vi "sort cycle unknown.vi"(6 "which order":string[](array[string])=["sequence number", "position", "seq total count", "seq total q", "seq unnormed ratio", "std total count", "std total pq", "std norm", "seq ratio", "seq ext error", "seq ext error(%)", "seq int error", "seq int error(%)", "seq error", "seq error(%)", "seq ext vs int"], 8 "error in":errorcluster) -> (0 "error out":errorcluster)   [LabVIEW 2016]
doc: "Takes a sample type and sorts by sequence"
uses:
  controls/data control cluster.ctl
  <vilib>/Analysis/baseanly.llb/Mean (DBL).vi
  <vilib>/Analysis/NI_AALBase.lvlib
panel:
  out "array w/ subset deleted":dbl[][][](array[numeric])
  out "cycle result header":string[](array[string])
  out "output array 2":dbl[][](array[numeric])
  out "element 2":i32
  out "output array":dbl[][](array[numeric])
  out "element":i32
  out "x/y 2":dbl
  out "x/y":dbl
  out "Cycle data by seq 4":dbl[][](array[numeric])
  out "Cycle data by seq 3":dbl[][](array[numeric])
  out "Array 3":bool[](array[boolean])
  out "Cycle data by seq 2":dbl[][][](array[numeric])
  out "DATA CLUSTER out 2":T1
  out "cycle results labels":string[](array[string])
  out "sequence result header 2":string[](array[string])
  out "Array 2":dbl[][](array[numeric])
  out "index of element":i32
  out "sequence  Result":dbl[][][](array[numeric])
  out "Final result header":string[][](array[string])
  out "DATA CLUSTER out":T1
  out "sequence result header":string[](array[string])
  out "Array":i32[](array[numeric])
  out "cycle results dbl 2":dbl[][](array[numeric])
  out "Cycle data by seq":dbl[][][](array[numeric])
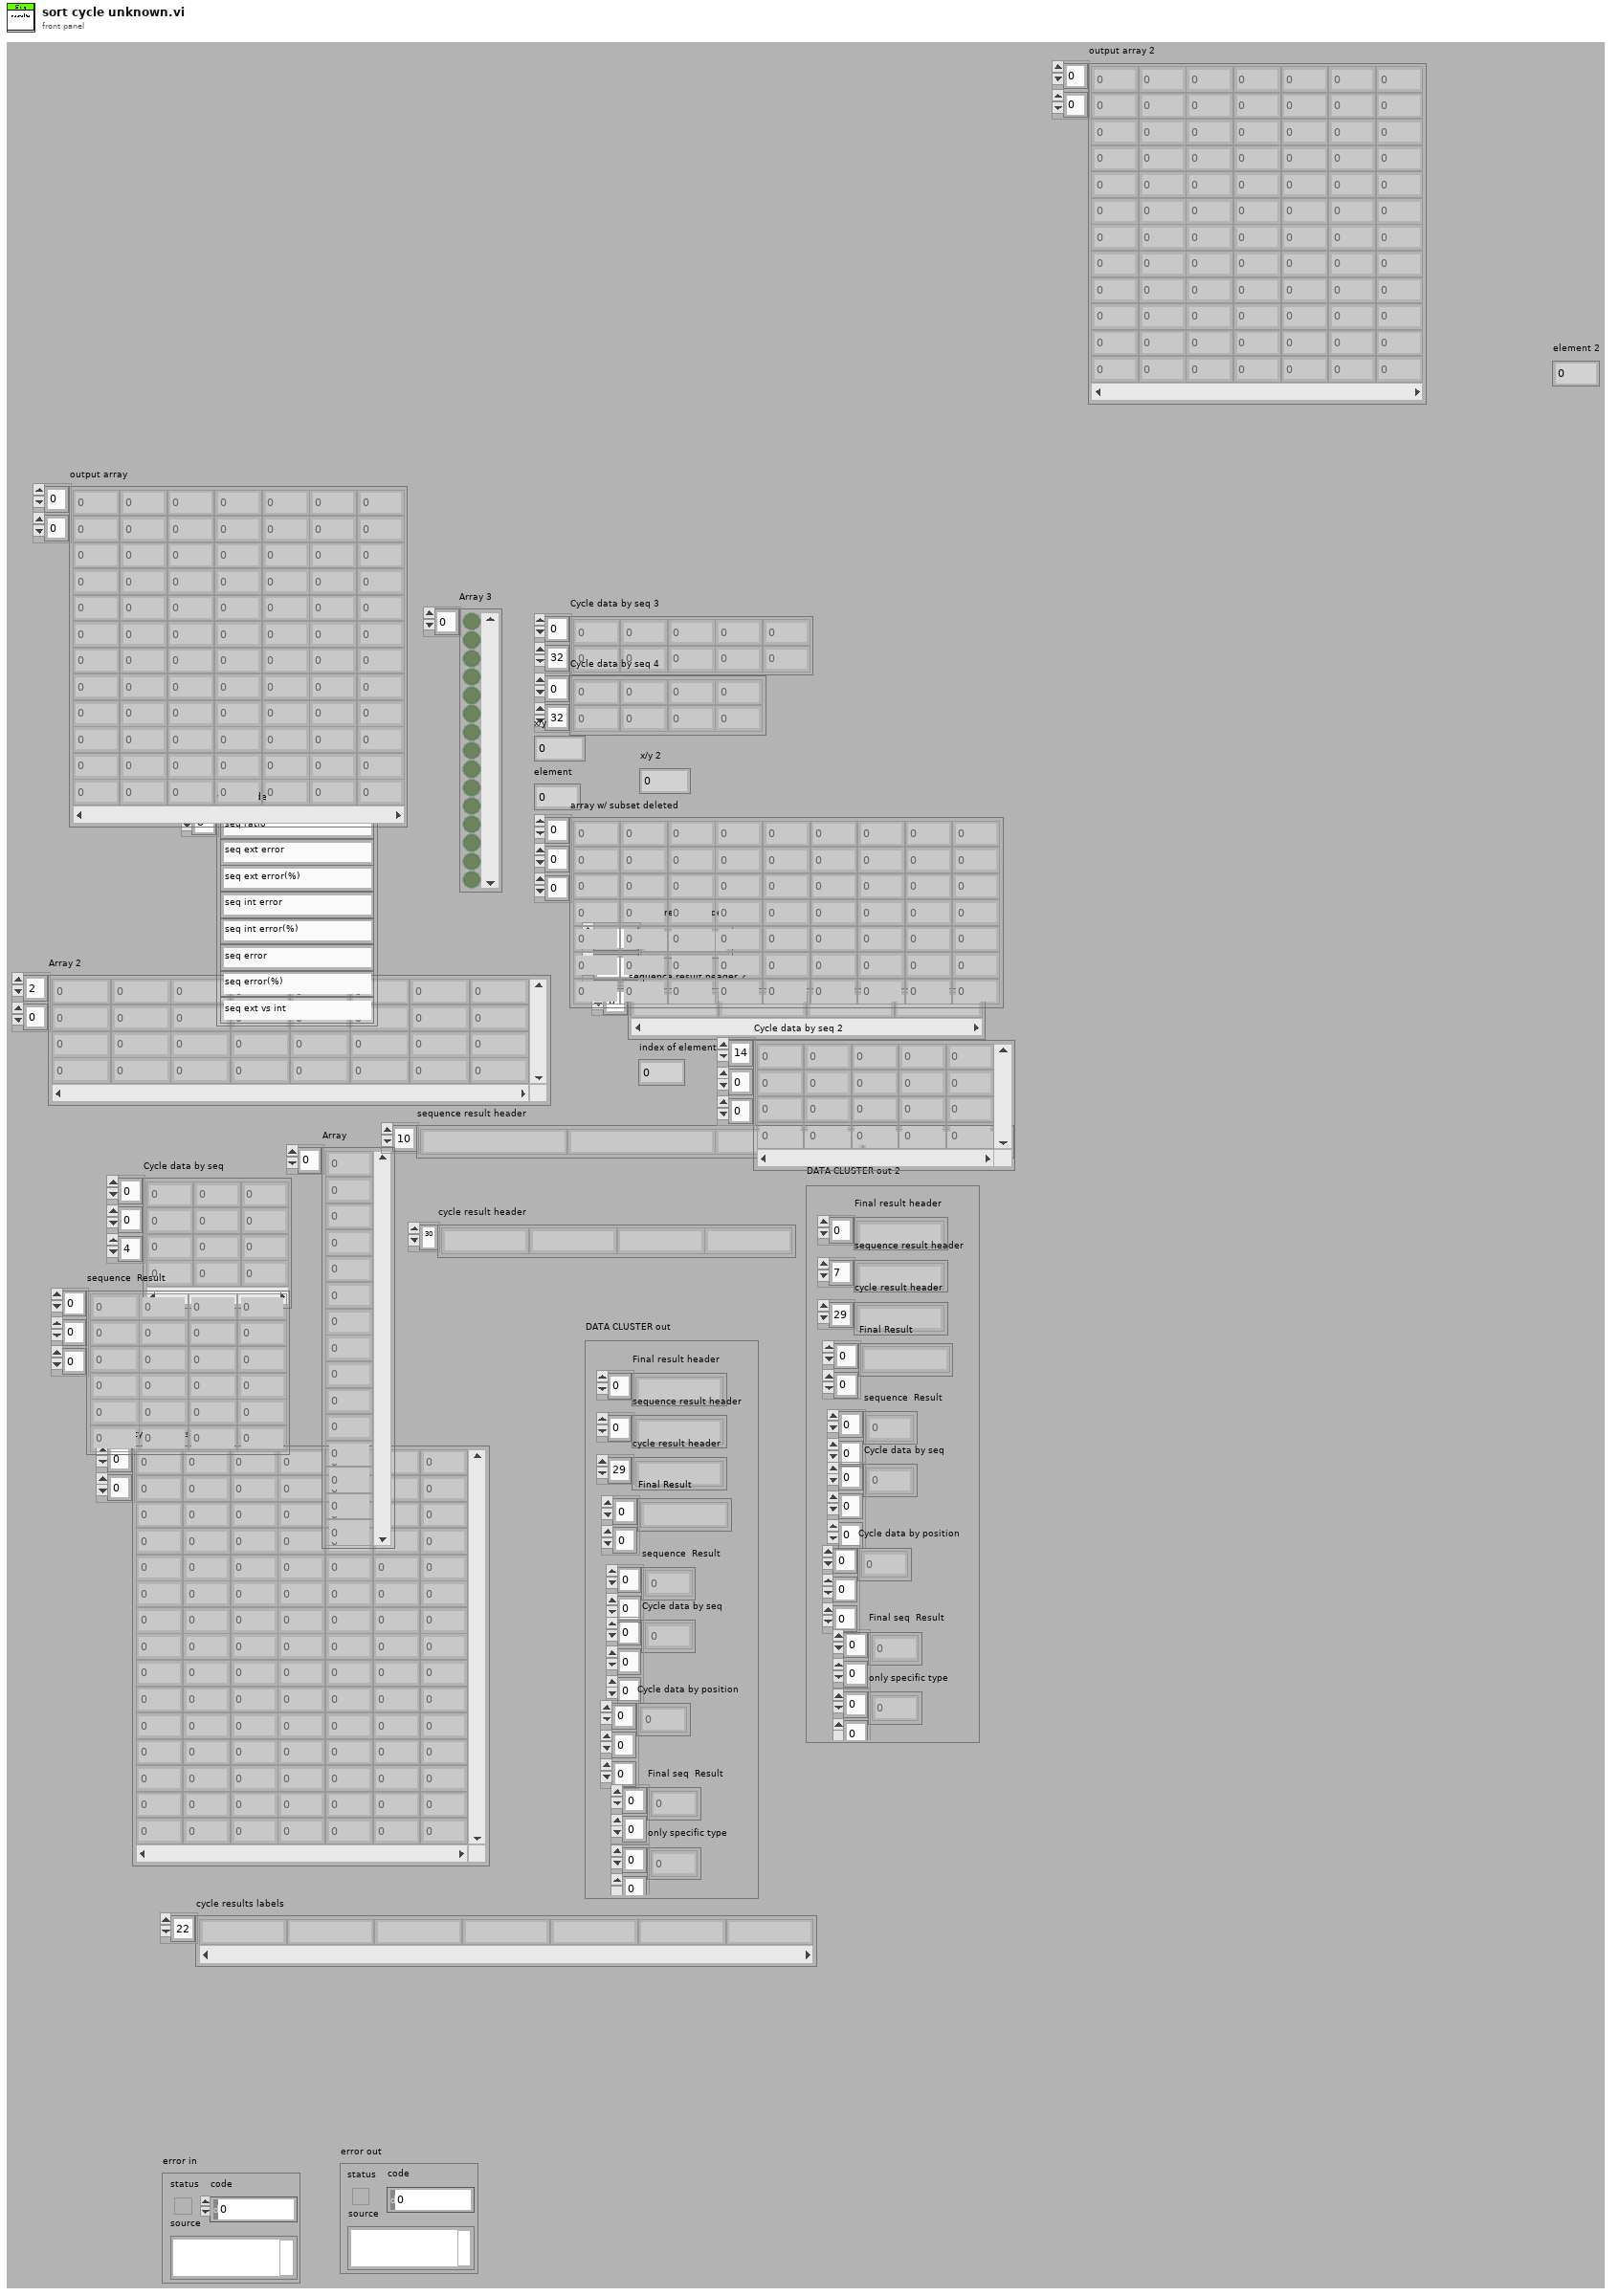
[diagram p1: front panel]
types:
  T1 = typedef "data control cluster.ctl" = cluster{"Final result header":string[], "sequence result header":string[], "cycle result header ":string[], "Final Result":string[][], "sequence  Result":dbl[][], "Cycle data by seq":dbl[][][], "Cycle data by position":dbl[][][], "Final seq  Result":dbl[][], "only specific type":dbl[][]}
  T2 = typedef "cycle results control.ctl" = cluster{"sample info":string[][], "cycle results labels":string[], "cycle results dbl":dbl[][]}
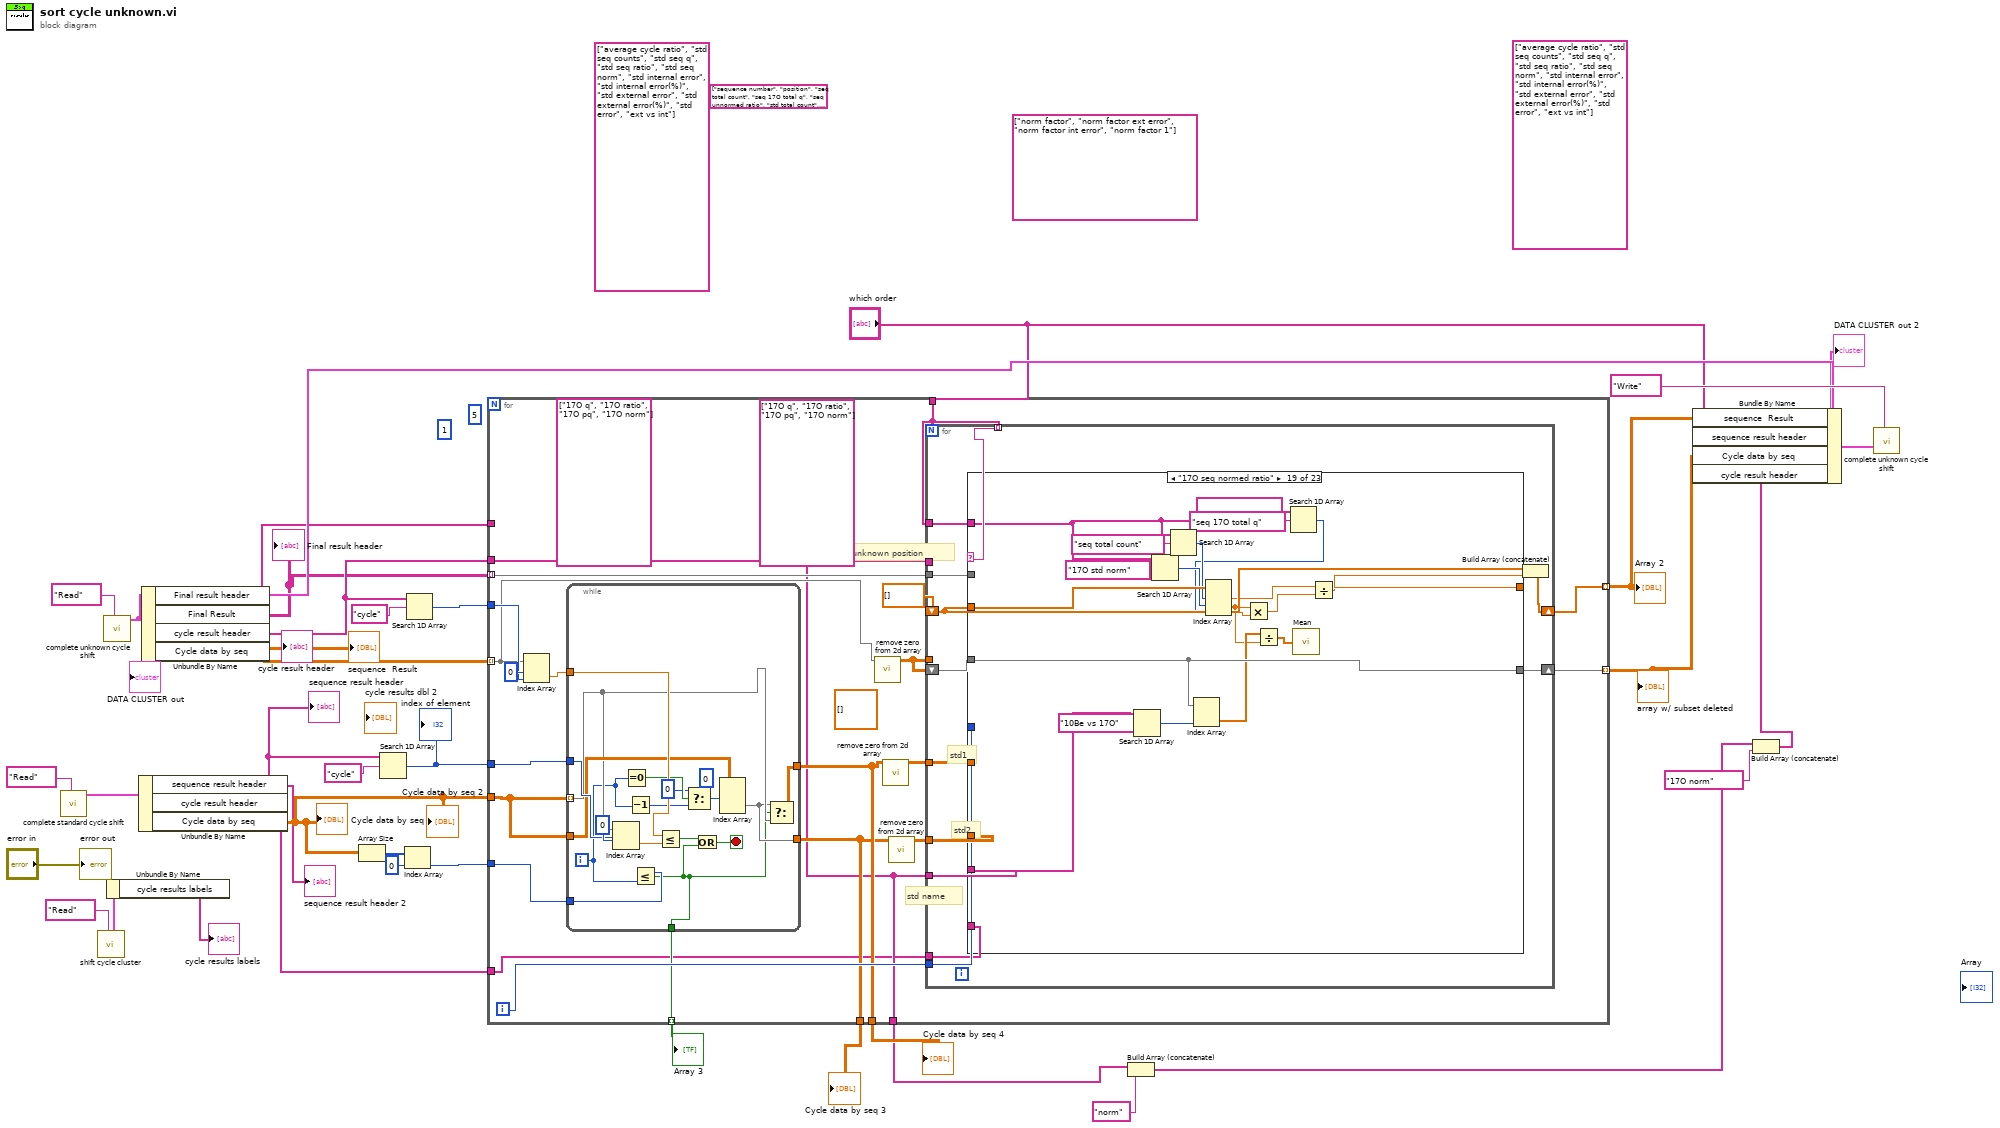
[diagram p0: block diagram]
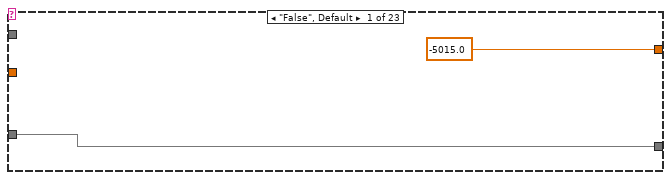
[diagram p2: hidden frame]
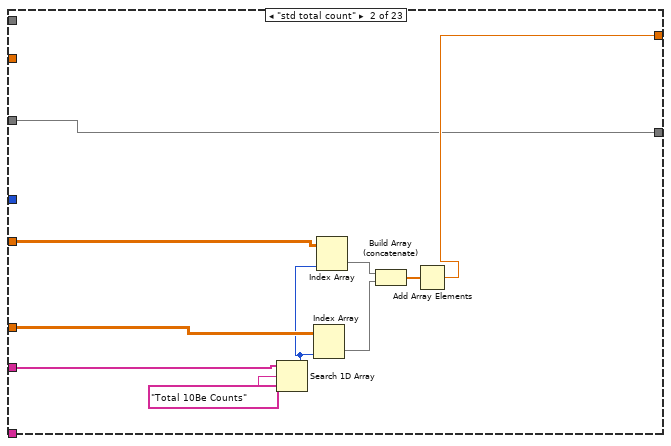
[diagram p3: hidden frame]
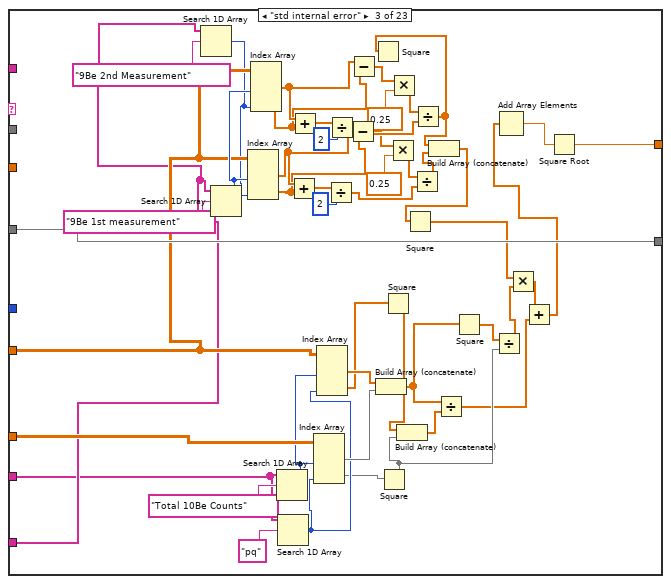
[diagram p4: hidden frame]
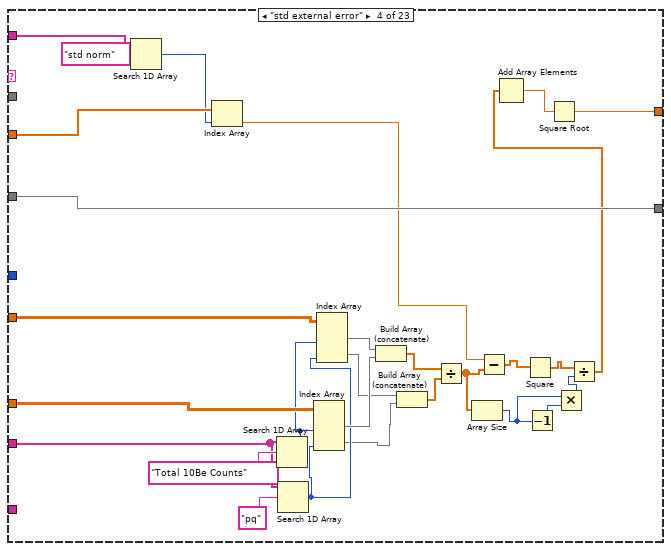
[diagram p5: hidden frame]
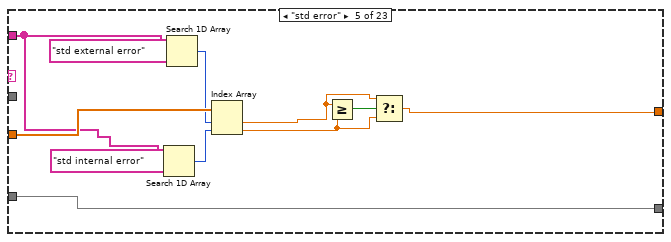
[diagram p6: hidden frame]
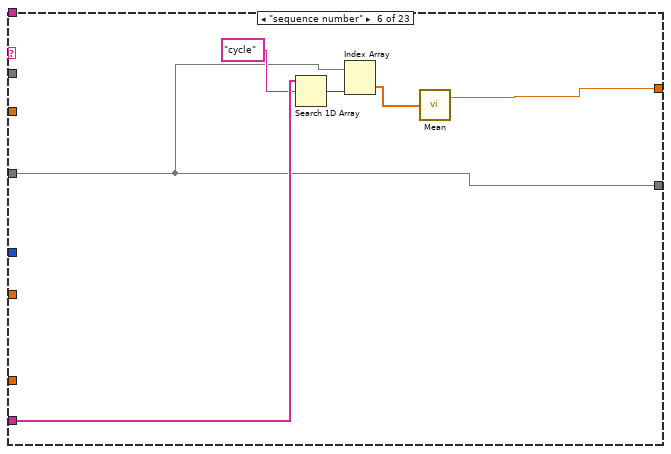
[diagram p7: hidden frame]
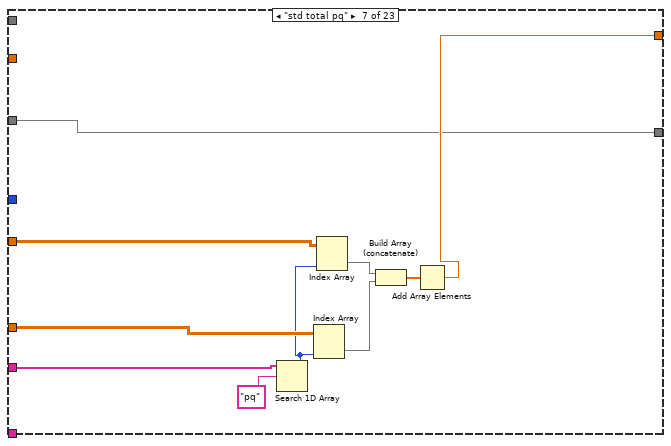
[diagram p8: hidden frame]
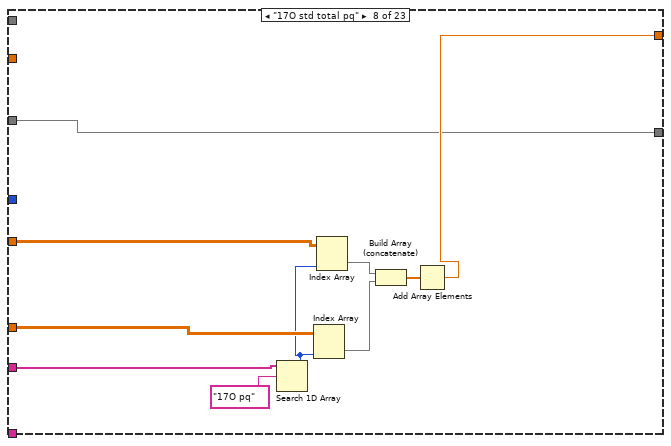
[diagram p9: hidden frame]
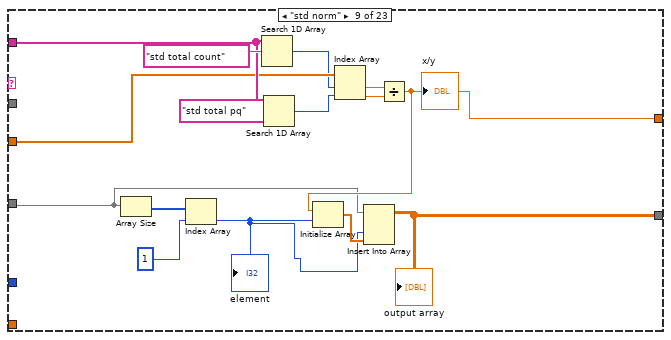
[diagram p10: hidden frame]
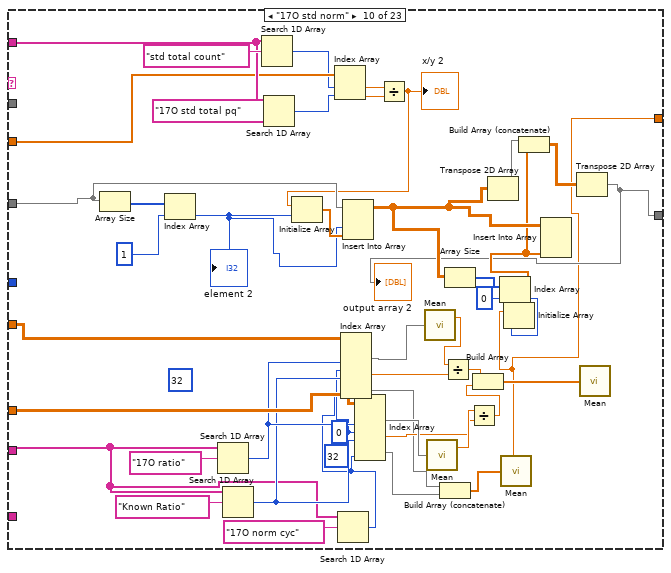
[diagram p11: hidden frame]
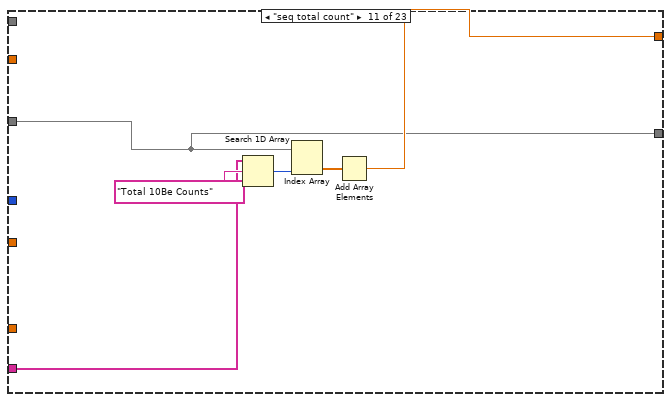
[diagram p12: hidden frame]
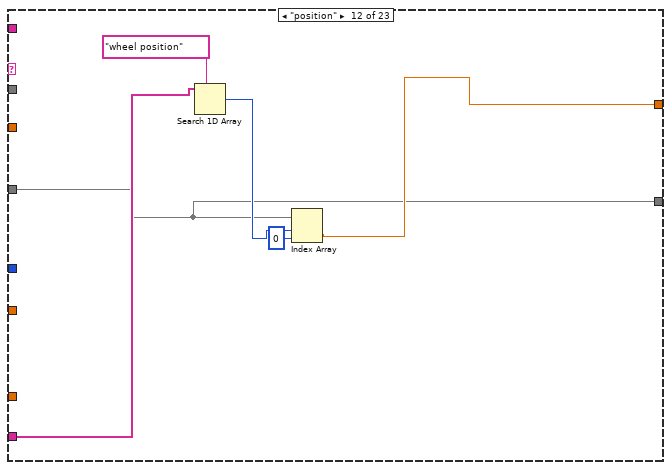
[diagram p13: hidden frame]
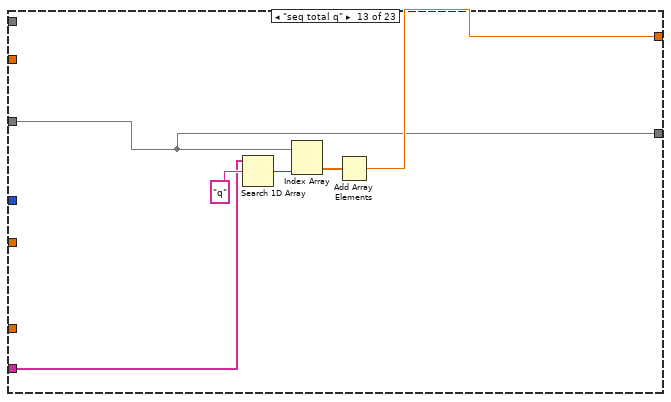
[diagram p14: hidden frame]
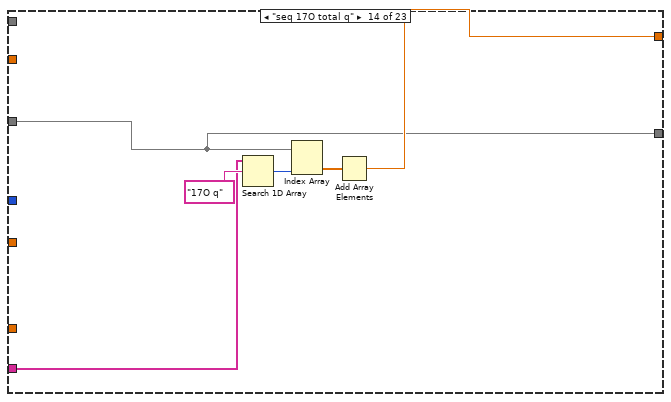
[diagram p15: hidden frame]
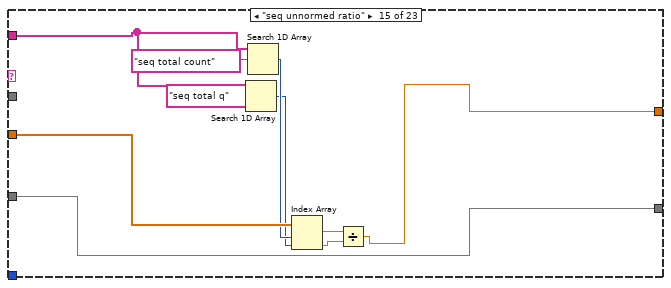
[diagram p16: hidden frame]
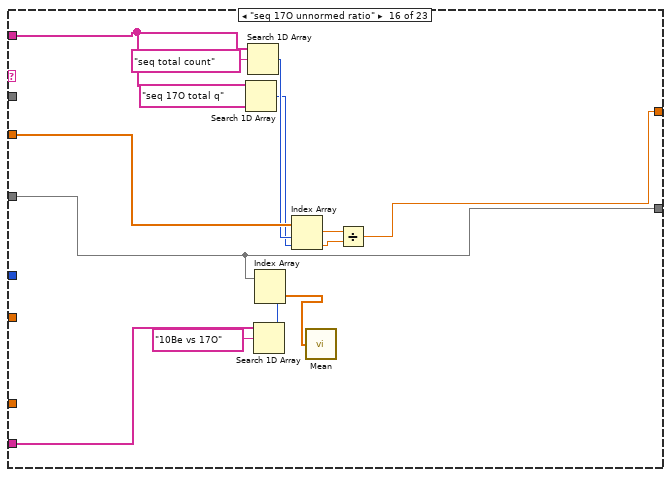
[diagram p17: hidden frame]
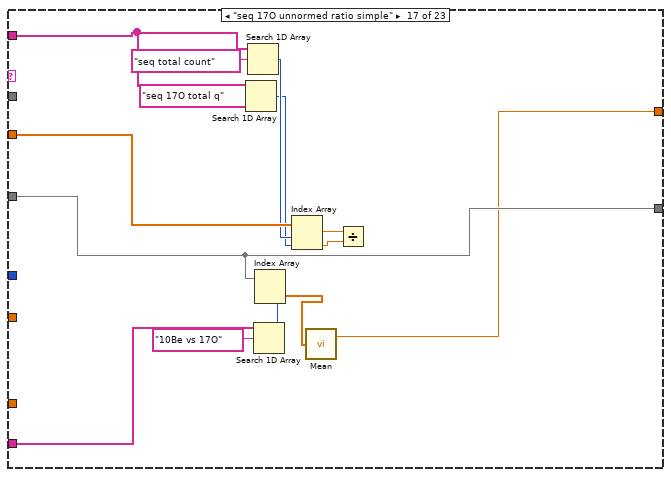
[diagram p18: hidden frame]
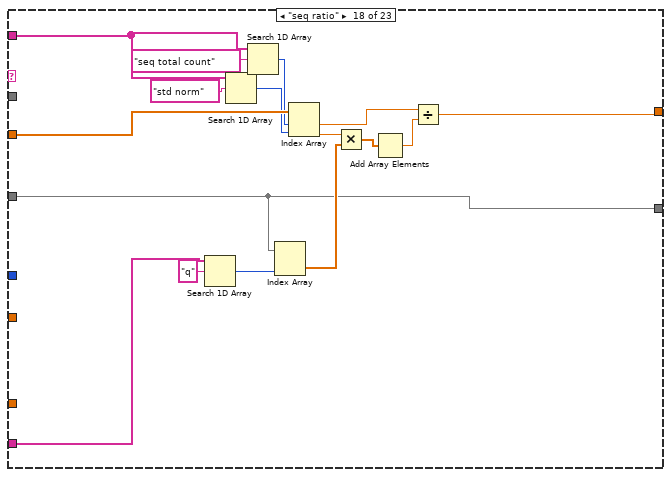
[diagram p19: hidden frame]
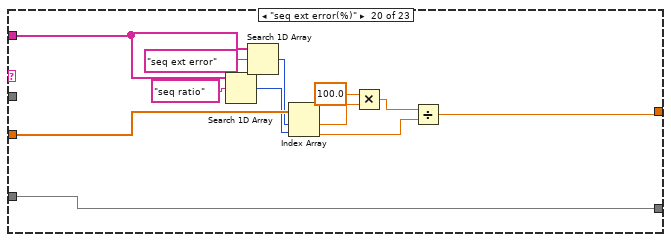
[diagram p20: hidden frame]
diagram:
  (unwired) 5
  (unwired) string[] ["average cycle ratio", "std seq counts", "std seq q", "std seq ratio", "std seq norm", "std internal error", "std internal error(%)", "std external error", "std external error(%)", "std error", "ext vs int"] ("which measurements")
  (unwired) string[] ["average cycle ratio", "std seq counts", "std seq q", "std seq ratio", "std seq norm", "std internal error", "std internal error(%)", "std external error", "std external error(%)", "std error", "ext vs int"] ("which measurements")
  (unwired) string[] ["sequence number", "position", "seq total count", "seq 17O total q", "seq unnormed ratio", "std total count", "17O std total pq", "std norm", "17O seq normed ratio", "17O seq external error", "17O seq ext error(%)", "seq int error", "seq int error(%)", "seq error", "seq error(%)", "seq ext vs int"] ("Array 5")
  (unwired) 1
  (unwired) string[] ["norm factor", "norm factor ext error", "norm factor int error", "norm factor 1"]
  n1 = call "complete standard cycle shift.vi"("read write shift"="Read") -> ("DATA CLUSTER out"=w31:T1)  [unwired: 9 in, 1 out]
  n2 = call "shift cycle cluster.vi"("read write shift"="Read") -> ("cycle results cluster out"=w20:T2)  [unwired: 9 in, 1 out]
  n3 = call "complete unknown cycle shift.vi"("read write shift"="Read") -> ("DATA CLUSTER out"=w17:T1)  [unwired: 9 in, 1 out]
  "DATA CLUSTER out" <- w17
  n4 = Unbundle By Name(w20) -> ("cycle results labels"=→"cycle results labels":string[])
  n5 = Unbundle By Name(w31) -> ("sequence result header"=→"sequence result header 2":string[], "cycle result header"=w23:string[], "Cycle data by seq"=w4:dbl[][][])
  "Cycle data by seq" <- w4
  "sequence result header" <- w23
  "Cycle data by seq 2" <- w4
  n6 = Unbundle By Name(w17) -> ("Final result header"=w10:string[], "Final Result"=w9:string[][], "cycle result header"=w14:string[], "Cycle data by seq"=w29:dbl[][][])
  "Final result header" <- w9
  "sequence  Result" <- w29
  "cycle result header" <- w14
  n7 = Array Size(array=w4) -> (size(s)=w27:i32[])
  n8 = Search 1D Array(1D array=w23, element="cycle") -> (index of element=w24:i32)  [unwired: 1 in]
  "index of element" <- w24
  n9 = Index Array(array=w27, index=0) -> (element=w25:i32)
  n10 = Search 1D Array(1D array=w14, element="cycle") -> (index of element=w28:i32)  [unwired: 1 in]
  n11 = for {
    tunnel: w29 -> [w45] mode=indexing
    tunnel: w4 -> [w51]
    tunnel: w28 -> [w55]
    tunnel: w25 -> [w54]
    tunnel: w24 -> [w52]
    tunnel: w23 -> [w36]
    tunnel: "which order" -> [w46]
    tunnel: w14 -> [w37]
    tunnel: [w48] -> w16 mode=indexing
    tunnel: [w43] -> w13 mode=indexing
    tunnel: [w42] -> w11
    tunnel: [w41] -> w12
    tunnel: w10 -> [_]
    tunnel: w9 -> [w40] mode=indexing
    tunnel: [w39] -> w7 mode=indexing
    tunnel: [w37] -> w6
    i -> [w44]
    (unwired) dbl[][] [] ("array w/ subset deleted")
    (unwired) string[] ["17O q", "17O ratio", "17O pq", "17O norm"] ("data requested")
    (unwired) string[] ["17O q", "17O ratio", "17O pq", "17O norm"] ("data requested")
    # "std name"
    # "std2"
    # "std1"
    # "unknown position"
    n12 = Index Array(array=w45, index (row)=0, index (col)=w55) -> (element=w53:dbl)
    n13 = while {
      tunnel: w54 -> [w436]
      tunnel: w53 -> [w433]
      tunnel: w51 -> [w428] mode=indexing
      tunnel: w52 -> [w434]
      tunnel: w51 -> [w429]
      tunnel: [w427] -> w41
      tunnel: [w426] -> w42
      tunnel: [w424] -> w43
      i -> [w421]
      stop <- w431 stop-if-true
      (unwired) 0 ("index (page)")
      n14 = Index Array(array=w428, index (row)=0, index (col)=w434) -> (element=w432:dbl)
      n15 = Equal To 0?(x=w421) -> (x = 0?=w423:bool)
      n16 = Decrement(x=w421) -> (x-1=w420:i32)
      n17 = Less Or Equal?(x=w436, y=w421) -> (x <= y?=w424:bool)
      n18 = Less Or Equal?(x=w433, y=w432) -> (x <= y?=w430:bool)
      n19 = Select(t=0, s=w423, f=w420) -> (s? t:f=w425:i32)
      n20 = Or(x=w430, y=w424) -> (x .or. y?=w431:bool)
      n21 = Index Array(array=w429, index (dim 0)=w425) -> (element=w427:dbl[][])  [unwired: 2 in]
      n22 = Select(t=w427, s=w424, f=w428) -> (s? t:f=w426:dbl[][])
    }
    n23 = call "remove zero from 2d array.vi"("Cycle data by seq"=w45) -> ("array w/ subset deleted"=w38:dbl[][])  [unwired: 10 in]
    n24 = call "remove zero from 2d array.vi"("Cycle data by seq"=w42) -> ("array w/ subset deleted"=w50:dbl[][])  [unwired: 10 in]
    n25 = call "remove zero from 2d array.vi"("Cycle data by seq"=w41) -> ("array w/ subset deleted"=w49:dbl[][])  [unwired: 10 in]
    n26 = for {
      tunnel: w37 -> [w69]
      tunnel: w46 -> [w68] mode=indexing
      tunnel: w50 -> [w67]
      tunnel: w49 -> [w66]
      tunnel: w37 -> [_]
      shift-right: [w57] -> w48
      shift-left: dbl[] [] ("Array 2") -> [w64]
      tunnel: w46 -> [w63]
      tunnel: w38 -> [_]
      tunnel: w44 -> [w62]
      tunnel: w40 -> [w61]
      shift-right: [w60] -> w39
      shift-left: w38 -> [w59]
      tunnel: w36 -> [w58]
      n27 = case shown="\"17O seq normed ratio\"" w68 {
        tunnel: w69 -> [_ w81 w98 w149 _ w174 w184 w194 _ w212 w259 w263 w271 w277 _ w290 w303 w328 w347 _ _ w393 w415]
        tunnel: w67 -> [_ w78 w121 w151 _ _ w181 w191 _ w237 _ _ _ _ _ _ _ _ _ _ _ _ _]
        tunnel: w66 -> [_ w79 w128 w156 _ _ w182 w192 _ w238 _ _ _ _ _ _ _ _ _ _ _ _ _]
        tunnel: [-5015.0 ("Numeric") w73 w82 w144 w158 w169 w176 w186 w199 w214 w256 w265 w268 w274 w280 w289 w304 w318 w339 w357 w369 w379 w401] -> w65
        tunnel: w64 -> [_ _ _ w140 w166 _ _ _ w206 w251 _ _ _ _ w287 w301 w315 w331 w350 w362 w374 w396 w418]
        tunnel: w63 -> [_ _ _ w142 w163 _ _ _ w208 w253 _ _ _ _ w285 w299 w313 w326 w336 w360 w372 w391 w413]
        tunnel: w59 -> [w70 w72 w124 w152 w168 w171 w175 w185 w198 w242 w255 w261 w267 w273 w279 w293 w307 w317 w343 w352 w364 w376 w398]
        tunnel: w62 -> [_ _ _ _ _ _ _ _ _ _ _ _ _ _ _ _ _ _ _ _ _ _ _]
        tunnel: w61 -> [_ _ _ _ _ _ _ _ _ _ _ _ _ _ _ _ _ _ _ _ _ _ _]
        tunnel: [w70 w72 w124 w152 w168 w171 w175 w185 w195 w217 w255 w261 w267 w273 w279 w293 w307 w317 w343 w352 w364 w376 w398] -> w60
        tunnel: w58 -> [_ _ w119 _ _ _ _ _ _ _ _ _ _ _ _ _ _ _ _ _ _ _ _]
        frame "False", Default {
        }
        frame "std total count" {
          n28 = Search 1D Array(1D array=w81, element="Total 10Be Counts") -> (index of element=w77:i32)  [unwired: 1 in]
          n29 = Index Array(array=w79, index (col)=w77) -> (element=w75:dbl[])  [unwired: 1 in]
          n30 = Index Array(array=w78, index (col)=w77) -> (element=w76:dbl[])  [unwired: 1 in]
          n31 = Build Array (concatenate)(w76, w75) -> (w74:dbl[])
          n32 = Add Array Elements(numeric array=w74) -> (sum=w73:dbl)
        }
        frame "std internal error" {
          n33 = Search 1D Array(1D array=w119, element="9Be 2nd Measurement") -> (index of element=w111:i32)  [unwired: 1 in]
          n34 = Search 1D Array(1D array=w119, element="9Be 1st measurement") -> (index of element=w123:i32)  [unwired: 1 in]
          n35 = Index Array(array=w121, index (col) #1=w123, index (col) #2=w111) -> (element #1=w103:dbl[], element #2=w102:dbl[])  [unwired: 2 in]
          n36 = Index Array(array=w121, index (col) #1=w123, index (col) #2=w111) -> (element #1=w117:dbl[], element #2=w110:dbl[])  [unwired: 2 in]
          n37 = Search 1D Array(1D array=w98, element="Total 10Be Counts") -> (index of element=w127:i32)  [unwired: 1 in]
          n38 = Search 1D Array(1D array=w98, element="pq") -> (index of element=w97:i32)  [unwired: 1 in]
          n39 = Add(x=w103, y=w102) -> (x+y=w104:dbl[])
          n40 = Add(x=w117, y=w110) -> (x+y=w118:dbl[])
          n41 = Index Array(array=w128, index (col) #1=w127, index (col) #2=w97) -> (element #1=w125:dbl[], element #2=w94:dbl[])  [unwired: 2 in]
          n42 = Index Array(array=w121, index (col) #1=w127, index (col) #2=w97) -> (element #1=w126:dbl[], element #2=w95:dbl[])  [unwired: 2 in]
          n43 = Divide(x=w104, y=2 ("Numeric")) -> (x/y=w108:dbl[])
          n44 = Divide(x=w118, y=2 ("Numeric")) -> (x/y=w113:dbl[])
          n45 = Subtract(x=w103, y=w102) -> (x-y=w107:dbl[])
          n46 = Subtract(x=w117, y=w110) -> (x-y=w114:dbl[])
          n47 = Build Array (concatenate)(w126, w125) -> (w91:dbl[])
          n48 = Square(x=w94) -> (x^2=w89:dbl[])
          n49 = Square(x=w95) -> (x^2=w93:dbl[])
          n50 = Multiply(x=w107, y=0.25 ("Numeric")) -> (x*y=w109:dbl[])
          n51 = Multiply(x=w114, y=0.25 ("Numeric")) -> (x*y=w112:dbl[])
          n52 = Build Array (concatenate)(w93, w89) -> (w92:dbl[])
          n53 = Divide(x=w109, y=w108) -> (x/y=w101:dbl[])
          n54 = Divide(x=w112, y=w113) -> (x/y=w100:dbl[])
          n55 = Square(x=w100) -> ()  [unwired: 1 out]
          n56 = Build Array (concatenate)(w100, w101) -> (w96:dbl[])
          n57 = Square(x=w96) -> (x^2=w88:dbl[])
          n58 = Divide(x=w91, y=w92) -> (x/y=w86:dbl[])
          n59 = Square(x=w91) -> (x^2=w90:dbl[])
          n60 = Divide(x=w90, y=w89) -> (x/y=w87:dbl[])
          n61 = Multiply(x=w88, y=w87) -> (x*y=w85:dbl[])
          n62 = Add(x=w85, y=w86) -> (x+y=w84:dbl[])
          n63 = Add Array Elements(numeric array=w84) -> (sum=w83:dbl)
          n64 = Square Root(x=w83) -> (sqrt(x)=w82:dbl)
        }
        frame "std external error" {
          n65 = Search 1D Array(1D array=w142, element="std norm") -> (index of element=w139:i32)  [unwired: 1 in]
          n66 = Index Array(array=w140, index=w139) -> (element=w137:dbl)
          n67 = Search 1D Array(1D array=w149, element="Total 10Be Counts") -> (index of element=w155:i32)  [unwired: 1 in]
          n68 = Search 1D Array(1D array=w149, element="pq") -> (index of element=w148:i32)  [unwired: 1 in]
          n69 = Index Array(array=w156, index (col) #1=w155, index (col) #2=w148) -> (element #1=w153:dbl[], element #2=w138:dbl[])  [unwired: 2 in]
          n70 = Index Array(array=w151, index (col) #1=w155, index (col) #2=w148) -> (element #1=w154:dbl[], element #2=w143:dbl[])  [unwired: 2 in]
          n71 = Build Array (concatenate)(w154, w153) -> (w146:dbl[])
          n72 = Build Array (concatenate)(w143, w138) -> (w147:dbl[])
          n73 = Divide(x=w146, y=w147) -> (x/y=w136:dbl[])
          n74 = Array Size(array=w136) -> (size(s)=w134:i32)
          n75 = Subtract(x=w137, y=w136) -> (x-y=w133:dbl[])
          n76 = Square(x=w133) -> (x^2=w132:dbl[])
          n77 = Decrement(x=w134) -> (x-1=w135:i32)
          n78 = Multiply(x=w134, y=w135) -> (x*y=w131:i32)
          n79 = Divide(x=w132, y=w131) -> (x/y=w130:dbl[])
          n80 = Add Array Elements(numeric array=w130) -> (sum=w145:dbl)
          n81 = Square Root(x=w145) -> (sqrt(x)=w144:dbl)
        }
        frame "std error" {
          n82 = Search 1D Array(1D array=w163, element="std internal error") -> (index of element=w162:i32)  [unwired: 1 in]
          n83 = Search 1D Array(1D array=w163, element="std external error") -> (index of element=w165:i32)  [unwired: 1 in]
          n84 = Index Array(array=w166, index #1=w165, index #2=w162) -> (element #1=w160:dbl, element #2=w159:dbl)
          n85 = Greater Or Equal?(x=w160, y=w159) -> (x >= y?=w161:bool)
          n86 = Select(t=w160, s=w161, f=w159) -> (s? t:f=w158:dbl)
        }
        frame "sequence number" {
          n87 = Search 1D Array(1D array=w174, element="cycle") -> (index of element=w172:i32)  [unwired: 1 in]
          n88 = Index Array(array=w171, index (col)=w172) -> (element=w170:dbl[])  [unwired: 1 in]
          n89 = call-poly <vilib>:"Mean.vi"("X"=w170) -> ("mean"=w169:dbl)  [unwired: 1 out]
        }
        frame "std total pq" {
          n90 = Search 1D Array(1D array=w184, element="pq") -> (index of element=w180:i32)  [unwired: 1 in]
          n91 = Index Array(array=w182, index (col)=w180) -> (element=w178:dbl[])  [unwired: 1 in]
          n92 = Index Array(array=w181, index (col)=w180) -> (element=w179:dbl[])  [unwired: 1 in]
          n93 = Build Array (concatenate)(w179, w178) -> (w177:dbl[])
          n94 = Add Array Elements(numeric array=w177) -> (sum=w176:dbl)
        }
        frame "17O std total pq" {
          n95 = Search 1D Array(1D array=w194, element="17O pq") -> (index of element=w190:i32)  [unwired: 1 in]
          n96 = Index Array(array=w192, index (col)=w190) -> (element=w188:dbl[])  [unwired: 1 in]
          n97 = Index Array(array=w191, index (col)=w190) -> (element=w189:dbl[])  [unwired: 1 in]
          n98 = Build Array (concatenate)(w189, w188) -> (w187:dbl[])
          n99 = Add Array Elements(numeric array=w187) -> (sum=w186:dbl)
        }
        frame "std norm" {
          n100 = Array Size(array=w198) -> (size(s)=w201:i32[])
          n101 = Index Array(array=w201, index=1) -> (element=w196:i32)
          "element" <- w196
          n102 = Search 1D Array(1D array=w208, element="std total count") -> (index of element=w205:i32)  [unwired: 1 in]
          n103 = Search 1D Array(1D array=w208, element="std total pq") -> (index of element=w204:i32)  [unwired: 1 in]
          n104 = Index Array(array=w206, index #1=w205, index #2=w204) -> (element #1=w202:dbl, element #2=w203:dbl)
          n105 = Divide(x=w202, y=w203) -> (x/y=w199:dbl)
          "x/y" <- w199
          n106 = Initialize Array(w199, w196) -> (w197:dbl[])
          n107 = Insert Into Array(array=w198, index (col)=w196, new element=w197) -> (w195:dbl[][])  [unwired: 1 in]
          "output array" <- w195
        }
        frame "17O std norm" {
          (unwired) 32 ("index (col)")
          (unwired) 32 ("index (col)")
          w234 = 0 ("disabled index (row)")
          n108 = Array Size(array=w242) -> (size(s)=w246:i32[])
          n109 = Index Array(array=w246, index=1) -> (element=w243:i32)
          "element 2" <- w243
          n110 = Search 1D Array(1D array=w212, element="17O ratio") -> (index of element=w236:i32)  [unwired: 1 in]
          n111 = Search 1D Array(1D array=w212, element="Known Ratio") -> (index of element=w235:i32)  [unwired: 1 in]
          n112 = Search 1D Array(1D array=w253, element="std total count") -> (index of element=w250:i32)  [unwired: 1 in]
          n113 = Search 1D Array(1D array=w253, element="17O std total pq") -> (index of element=w249:i32)  [unwired: 1 in]
          n114 = Index Array(array=w251, index #1=w250, index #2=w249) -> (element #1=w247:dbl, element #2=w248:dbl)
          n115 = Search 1D Array(1D array=w212, element="17O norm cyc") -> (index of element=w211:i32)  [unwired: 1 in]
          n116 = Index Array(array=w237, index (col) #1=w236, index (row) #2=w234, index (col) #2=w235, index (col) #3=w211) -> (element #1=w233:dbl[], element #2=w231:dbl, element #3=w216:dbl[])  [unwired: 2 in]
          n117 = Index Array(array=w238, index (col) #1=w236, index (row) #2=w234, index (col) #2=w235, index (col) #3=w211) -> (element #1=w230:dbl[], element #2=w228:dbl, element #3=w215:dbl[])  [unwired: 2 in]
          n118 = Divide(x=w247, y=w248) -> (x/y=w241:dbl)
          "x/y 2" <- w241
          n119 = Initialize Array(w241, w243) -> (w244:dbl[])
          n120 = Insert Into Array(array=w242, index (col)=w243, new element=w244) -> (w221:dbl[][])  [unwired: 1 in]
          n121 = call-poly <vilib>:"Mean.vi"("X"=w233) -> ("mean"=w232:dbl)  [unwired: 1 out]
          n122 = call-poly <vilib>:"Mean.vi"("X"=w230) -> ("mean"=w229:dbl)  [unwired: 1 out]
          n123 = Build Array (concatenate)(w216, w215) -> (w210:dbl[])
          n124 = Divide(x=w232, y=w231) -> (x/y=w226:dbl)
          n125 = Array Size(array=w221) -> (size(s)=w224:i32[])
          n126 = Divide(x=w229, y=w228) -> (x/y=w227:dbl)
          n127 = Build Array(w226, w227) -> (w225:dbl[])
          n128 = Transpose 2D Array(2D array=w221) -> (transposed array=w220:dbl[][])
          n129 = Index Array(array=w224, index=0) -> (element=w223:i32)
          n130 = call-poly <vilib>:"Mean.vi"("X"=w210) -> ("mean"=w214:dbl)  [unwired: 1 out]
          n131 = Initialize Array(w214, w223) -> (w219:dbl[])
          n132 = Build Array (concatenate)(w220, w219) -> (w218:dbl[][])
          n133 = Insert Into Array(array=w221, new element=w219) -> ()  [unwired: 2 in, 1 out]
          n134 = Transpose 2D Array(2D array=w218) -> (transposed array=w217:dbl[][])
          "output array 2" <- w217
          n135 = call-poly <vilib>:"Mean.vi"("X"=w225) -> ()  [unwired: 2 out]
        }
        frame "seq total count" {
          n136 = Search 1D Array(1D array=w259, element="Total 10Be Counts") -> (index of element=w258:i32)  [unwired: 1 in]
          n137 = Index Array(array=w255, index (col)=w258) -> (element=w257:dbl[])  [unwired: 1 in]
          n138 = Add Array Elements(numeric array=w257) -> (sum=w256:dbl)
        }
        frame "position" {
          n139 = Search 1D Array(1D array=w263, element="wheel position") -> (index of element=w264:i32)  [unwired: 1 in]
          n140 = Index Array(array=w261, index (row)=w264, index (col)=0 ("disabled index (col)")) -> (element=w265:dbl)
        }
        frame "seq total q" {
          n141 = Search 1D Array(1D array=w271, element="q") -> (index of element=w270:i32)  [unwired: 1 in]
          n142 = Index Array(array=w267, index (col)=w270) -> (element=w269:dbl[])  [unwired: 1 in]
          n143 = Add Array Elements(numeric array=w269) -> (sum=w268:dbl)
        }
        frame "seq 17O total q" {
          n144 = Search 1D Array(1D array=w277, element="17O q") -> (index of element=w276:i32)  [unwired: 1 in]
          n145 = Index Array(array=w273, index (col)=w276) -> (element=w275:dbl[])  [unwired: 1 in]
          n146 = Add Array Elements(numeric array=w275) -> (sum=w274:dbl)
        }
        frame "seq unnormed ratio" {
          n147 = Search 1D Array(1D array=w285, element="seq total q") -> (index of element=w283:i32)  [unwired: 1 in]
          n148 = Search 1D Array(1D array=w285, element="seq total count") -> (index of element=w286:i32)  [unwired: 1 in]
          n149 = Index Array(array=w287, index #1=w286, index #2=w283) -> (element #1=w281:dbl, element #2=w282:dbl)
          n150 = Divide(x=w281, y=w282) -> (x/y=w280:dbl)
        }
        frame "seq 17O unnormed ratio" {
          n151 = Search 1D Array(1D array=w299, element="seq 17O total q") -> (index of element=w297:i32)  [unwired: 1 in]
          n152 = Search 1D Array(1D array=w299, element="seq total count") -> (index of element=w300:i32)  [unwired: 1 in]
          n153 = Search 1D Array(1D array=w290, element="10Be vs 17O") -> (index of element=w292:i32)  [unwired: 1 in]
          n154 = Index Array(array=w293, index (col)=w292) -> (element=w291:dbl[])  [unwired: 1 in]
          n155 = Index Array(array=w301, index #1=w300, index #2=w297) -> (element #1=w295:dbl, element #2=w296:dbl)
          n156 = call-poly <vilib>:"Mean.vi"("X"=w291) -> ()  [unwired: 2 out]
          n157 = Divide(x=w295, y=w296) -> (x/y=w289:dbl)
        }
        frame "seq 17O unnormed ratio simple" {
          n158 = Search 1D Array(1D array=w313, element="seq 17O total q") -> (index of element=w311:i32)  [unwired: 1 in]
          n159 = Search 1D Array(1D array=w313, element="seq total count") -> (index of element=w314:i32)  [unwired: 1 in]
          n160 = Search 1D Array(1D array=w303, element="10Be vs 17O") -> (index of element=w306:i32)  [unwired: 1 in]
          n161 = Index Array(array=w307, index (col)=w306) -> (element=w305:dbl[])  [unwired: 1 in]
          n162 = Index Array(array=w315, index #1=w314, index #2=w311) -> (element #1=w309:dbl, element #2=w310:dbl)
          n163 = call-poly <vilib>:"Mean.vi"("X"=w305) -> ("mean"=w304:dbl)  [unwired: 1 out]
          n164 = Divide(x=w309, y=w310) -> ()  [unwired: 1 out]
        }
        frame "seq ratio" {
          n165 = Search 1D Array(1D array=w328, element="q") -> (index of element=w327:i32)  [unwired: 1 in]
          n166 = Search 1D Array(1D array=w326, element="std norm") -> (index of element=w324:i32)  [unwired: 1 in]
          n167 = Search 1D Array(1D array=w326, element="seq total count") -> (index of element=w330:i32)  [unwired: 1 in]
          n168 = Index Array(array=w317, index (col)=w327) -> (element=w322:dbl[])  [unwired: 1 in]
          n169 = Index Array(array=w331, index #1=w330, index #2=w324) -> (element #1=w321:dbl, element #2=w323:dbl)
          n170 = Multiply(x=w323, y=w322) -> (x*y=w320:dbl[])
          n171 = Add Array Elements(numeric array=w320) -> (sum=w319:dbl)
          n172 = Divide(x=w321, y=w319) -> (x/y=w318:dbl)
        }
        frame "17O seq normed ratio" {
          n173 = Search 1D Array(1D array=w347, element="10Be vs 17O") -> (index of element=w346:i32)  [unwired: 1 in]
          n174 = Search 1D Array(1D array=w336, element="17O std norm") -> (index of element=w344:i32)  [unwired: 1 in]
          n175 = Search 1D Array(1D array=w336, element="seq total count") -> (index of element=w349:i32)  [unwired: 1 in]
          n176 = Index Array(array=w343, index (col)=w346) -> (element=w342:dbl[])  [unwired: 1 in]
          n177 = Search 1D Array(1D array=w336, element="seq 17O total q") -> (index of element=w335:i32)  [unwired: 1 in]
          n178 = Index Array(array=w350, index #1=w349, index #2=w344, index #3=w335) -> (element #1=w340:dbl, element #2=w338:dbl, element #3=w334:dbl)
          n179 = Multiply(x=w338, y=w334) -> (x*y=w333:dbl)
          n180 = Divide(x=w342, y=w338) -> (x/y=w341:dbl[])
          n181 = call-poly <vilib>:"Mean.vi"("X"=w341) -> ()  [unwired: 2 out]
          n182 = Divide(x=w340, y=w333) -> (x/y=w339:dbl)
        }
        frame "seq ext error(%)" {
          n183 = Search 1D Array(1D array=w360, element="seq ratio") -> (index of element=w358:i32)  [unwired: 1 in]
          n184 = Search 1D Array(1D array=w360, element="seq ext error") -> (index of element=w361:i32)  [unwired: 1 in]
          n185 = Index Array(array=w362, index #1=w361, index #2=w358) -> (element #1=w355:dbl, element #2=w356:dbl)
          n186 = Multiply(x=100.0, y=w355) -> (x*y=w353:dbl)
          n187 = Divide(x=w353, y=w356) -> (x/y=w357:dbl)
        }
        frame "17O seq ext error(%)" {
          n188 = Search 1D Array(1D array=w372, element="17O seq normed ratio") -> (index of element=w370:i32)  [unwired: 1 in]
          n189 = Search 1D Array(1D array=w372, element="17O seq external error") -> (index of element=w373:i32)  [unwired: 1 in]
          n190 = Index Array(array=w374, index #1=w373, index #2=w370) -> (element #1=w367:dbl, element #2=w368:dbl)
          n191 = Multiply(x=100.0, y=w367) -> (x*y=w365:dbl)
          n192 = Divide(x=w365, y=w368) -> (x/y=w369:dbl)
        }
        frame "seq ext error" {
          n193 = Search 1D Array(1D array=w393, element="ratio") -> (index of element=w392:i32)  [unwired: 1 in]
          n194 = Search 1D Array(1D array=w391, element="std norm") -> (index of element=w389:i32)  [unwired: 1 in]
          n195 = Search 1D Array(1D array=w391, element="seq ratio") -> (index of element=w395:i32)  [unwired: 1 in]
          n196 = Index Array(array=w376, index (col)=w392) -> (element=w384:dbl[])  [unwired: 1 in]
          n197 = Index Array(array=w396, index #1=w395, index #2=w389) -> (element #1=w386:dbl, element #2=w388:dbl)
          n198 = Divide(x=w384, y=w388) -> (x/y=w387:dbl[])
          n199 = Array Size(array=w384) -> (size(s)=w383:i32)
          n200 = Subtract(x=w386, y=w387) -> (x-y=w385:dbl[])
          n201 = Decrement(x=w383) -> (x-1=w382:i32)
          n202 = Multiply(x=w382, y=w383) -> (x*y=w381:i32)
          n203 = Square(x=w385) -> (x^2=w378:dbl[])
          n204 = Add Array Elements(numeric array=w378) -> (sum=w377:dbl)
          n205 = Divide(x=w377, y=w381) -> (x/y=w380:dbl)
          n206 = Square Root(x=w380) -> (sqrt(x)=w379:dbl)
        }
        frame "17O seq external error" {
          n207 = Search 1D Array(1D array=w415, element="17O ratio") -> (index of element=w414:i32)  [unwired: 1 in]
          n208 = Search 1D Array(1D array=w413, element="17O std norm") -> (index of element=w411:i32)  [unwired: 1 in]
          n209 = Search 1D Array(1D array=w413, element="17O seq normed ratio") -> (index of element=w417:i32)  [unwired: 1 in]
          n210 = Index Array(array=w398, index (col)=w414) -> (element=w406:dbl[])  [unwired: 1 in]
          n211 = Index Array(array=w418, index #1=w417, index #2=w411) -> (element #1=w408:dbl, element #2=w410:dbl)
          n212 = Divide(x=w406, y=w410) -> (x/y=w409:dbl[])
          n213 = Array Size(array=w406) -> (size(s)=w405:i32)
          n214 = Subtract(x=w408, y=w409) -> (x-y=w407:dbl[])
          n215 = Decrement(x=w405) -> (x-1=w404:i32)
          n216 = Multiply(x=w404, y=w405) -> (x*y=w403:i32)
          n217 = Square(x=w407) -> (x^2=w400:dbl[])
          n218 = Add Array Elements(numeric array=w400) -> (sum=w399:dbl)
          n219 = Divide(x=w399, y=w403) -> (x/y=w402:dbl)
          n220 = Square Root(x=w402) -> (sqrt(x)=w401:dbl)
        }
      }
      n221 = Build Array (concatenate)(w64, w65) -> (w57:dbl[])
    }
  }
  "Array 2" <- w16
  "Array 3" <- w13
  "Cycle data by seq 3" <- w12
  "Cycle data by seq 4" <- w11
  "array w/ subset deleted" <- w7
  n222 = Build Array (concatenate)(w6, "norm" ("String")) -> (w3:string[])
  n223 = Build Array (concatenate)(w3, "17O norm" ("String")) -> (w1:string[])
  n224 = Bundle By Name(cluster=w17, "sequence  Result"=w16, "sequence result header"="which order", "Cycle data by seq"=w7, "cycle result header"=w1) -> (w15:T1)
  "DATA CLUSTER out 2" <- w15
  n225 = call "complete unknown cycle shift.vi"("read write shift"="Write", "DATA CLUSTER in"=w15) -> ()  [unwired: 8 in, 2 out]
  "error out" <- "error in"
